vi "Get Available Data Sources.vi"(8 "error in (no error)":errorcluster) -> (0 "error out":errorcluster, 2 "Data Source Type":string[](array[string]), 3 "Data Sources":string[](array[string]))   [LabVIEW 2018, in "Database.lvlib"]
uses:
  Database.lvlib
  <vilib>/registry/registry.llb/Registry RtKey.ctl
  <vilib>/registry/registry.llb/Registry SAM.ctl
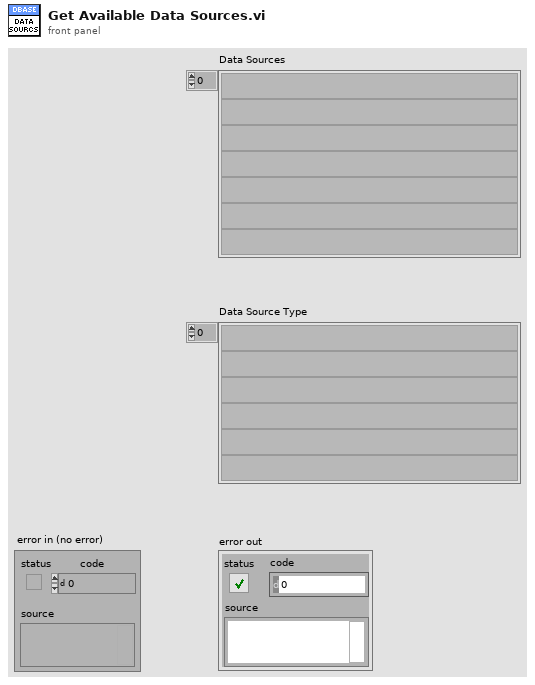
[diagram p1: front panel]
types:
  T1 = typedef "Registry SAM.ctl" = enum32{"KEY_QUERY_VALUE", "KEY_SET_VALUE", "KEY_CREATE_SUB_KEY", "KEY_ENUMERATE_SUB_KEYS", "KEY_NOTIFY", "KEY_CREATE_LINK", "KEY_READ", "KEY_WRITE", "KEY_ALL_ACCESS", "KEY_READ | KEY_WRITE"}
  T2 = typedef "Registry RtKey.ctl" = enum32{"HKEY_CLASSES_ROOT", "HKEY_CURRENT_USER", "HKEY_LOCAL_MACHINE", "HKEY_USERS", "HKEY_PERFORMANCE_DATA", "HKEY_CURRENT_CONFIG", "HKEY_DYN_DATA"}
  T3 = typedef "Registry refnum.ctl" = refnum<k1>
  T4 = cluster{"numValues":i32, "maxValueNameLen":i32, "maxValueDataLen":i32}
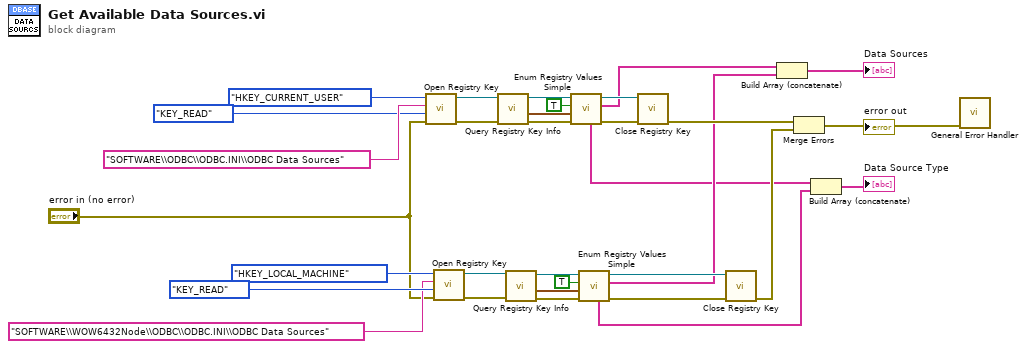
[diagram p0: block diagram]
diagram:
  n1 = call <vilib>:"Open Registry Key.vi"("error in (no error)"="error in (no error)", "security access mask (KEY_READ | KEY_WRITE)"=Registry_SAM."KEY_READ", "subkey"="SOFTWARE\\ODBC\\ODBC.INI\\ODBC Data Sources", "root key (HKEY_LOCAL_MACHINE)"=Registry_RtKey."HKEY_CURRENT_USER") -> ("error out"=w31:errorcluster, "refnum out"=w24:T3)  [unwired: 6 in]
  n2 = call <vilib>:"Open Registry Key.vi"("error in (no error)"="error in (no error)", "security access mask (KEY_READ | KEY_WRITE)"=Registry_SAM."KEY_READ", "subkey"="SOFTWARE\\WOW6432Node\\ODBC\\ODBC.INI\\ODBC Data Sources", "root key (HKEY_LOCAL_MACHINE)"=Registry_RtKey."HKEY_LOCAL_MACHINE") -> ("error out"=w10:errorcluster, "refnum out"=w9:T3)  [unwired: 6 in]
  n3 = call <vilib>:"Query Registry Key Info.vi"("error in (no error)"=w31, "refnum"=w24) -> ("error out"=w25:errorcluster, "value info"=w22:T4, "refnum out"=w23:T3)  [unwired: 5 in, 2 out]
  n4 = call <vilib>:"Query Registry Key Info.vi"("error in (no error)"=w10, "refnum"=w9) -> ("error out"=w13:errorcluster, "value info"=w15:T4, "refnum out"=w14:T3)  [unwired: 5 in, 2 out]
  n5 = call <vilib>:"Enum Registry Values Simple.vi"("error in (no error)"=w25, "value info"=w22, "retrieve data? (F)"=TRUE, "refnum"=w23) -> ("error out"=w32:errorcluster, "values"=w21:string[], "refnum out"=w30:T3, "String/Binary data"=w4:string[])  [unwired: 2 in, 2 out]
  n6 = call <vilib>:"Enum Registry Values Simple.vi"("error in (no error)"=w13, "value info"=w15, "retrieve data? (F)"=TRUE, "refnum"=w14) -> ("error out"=w11:errorcluster, "values"=w5:string[], "refnum out"=w12:T3, "String/Binary data"=w3:string[])  [unwired: 2 in, 2 out]
  n7 = call <vilib>:"Close Registry Key.vi"("error in (no error)"=w32, "refnum"=w30) -> ("error out"=w26:errorcluster)  [unwired: 5 in]
  n8 = call <vilib>:"Close Registry Key.vi"("error in (no error)"=w11, "refnum"=w12) -> ("error out"=w7:errorcluster)  [unwired: 5 in]
  n9 = Build Array (concatenate)(w21, w5) -> (→"Data Sources":string[])
  n10 = Merge Errors(w26, w7) -> (w8:errorcluster)
  "error out" <- w8
  n11 = Build Array (concatenate)(w4, w3) -> (→"Data Source Type":string[])
  n12 = call <vilib>:"General Error Handler.vi"("error in (no error)"=w8) -> ()  [unwired: 10 in, 5 out]
